vi "my_comands.vi"() -> ()   [LabVIEW 2018]
uses:
  <vilib>/Instr/_visa.llb/VISA Configure Serial Port (Instr).vi
panel:
  out "CRC16":string
  out "String":string
  in  "Array":u8[](array[numeric])=[97, 106, 241, 1, 0] format="%.0x"
  out "error out":errorcluster
  in  "baud rate (9600)":u32=9600
  in  "error in (no error)":errorcluster
  in  "VISA resource name":refnum<visa-resource-name>
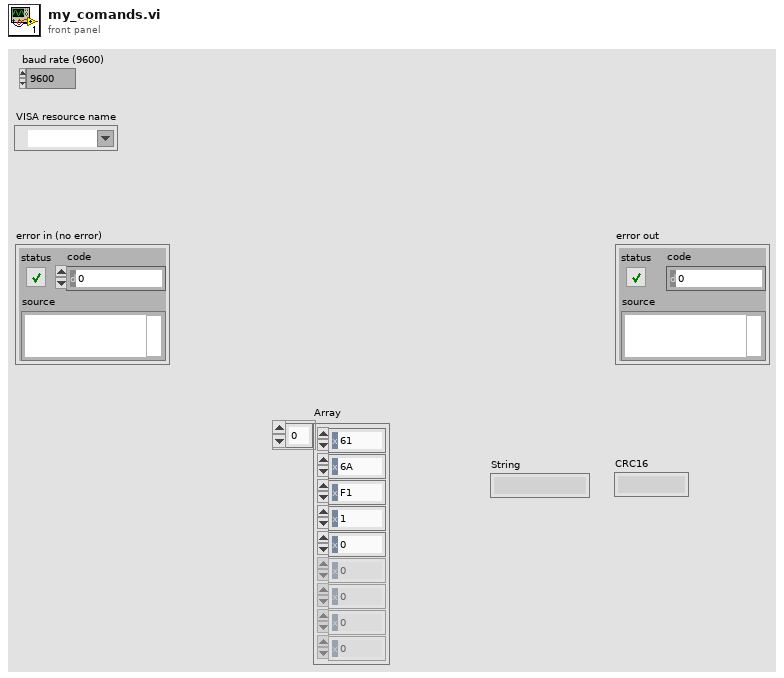
[diagram p1: front panel]
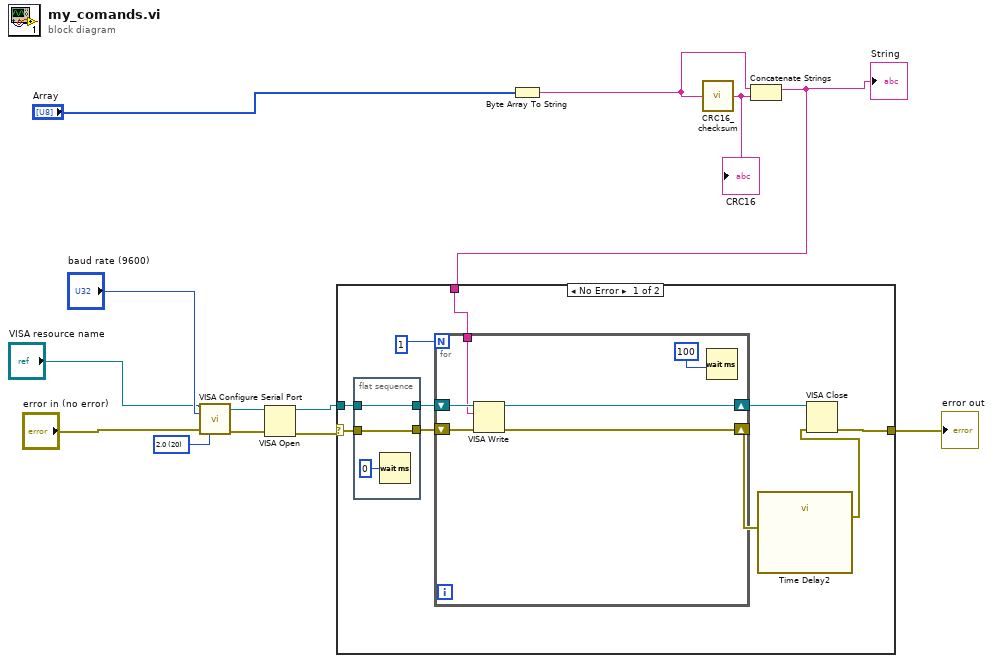
[diagram p0: block diagram]
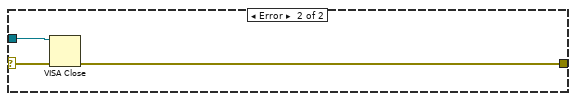
[diagram p2: hidden frame]
diagram:
  w1 = u16 20 items=["1.0"=10, "1.5"=15, "2.0"=20] ("stop bits (10: 1 bit)")
  n1 = call-poly "VISA Configure Serial Port"("VISA resource name"="VISA resource name", "baud rate (9600)"="baud rate (9600)", "error in (no error)"="error in (no error)", "stop bits (10: 1 bit)"=w1) -> ("VISA resource name out"=w3:refnum<visa-resource-name>, "error out"=w2:errorcluster)  [unwired: 10 in]
  n2 = VISA Open(error in (no error)=w2, VISA resource name=w3) -> (VISA resource name=w5:refnum<visa-resource-name>, error out=w4:errorcluster)  [unwired: 3 in]
  n3 = Byte Array To String(unsigned byte array="Array") -> (string=w8:string)
  n4 = call "CRC16_checksum.vi"("message"=w8) -> ("CRC16"=w10:string)
  "CRC16" <- w10
  n5 = Concatenate Strings(w8, w10) -> (w11:string)
  "String" <- w11
  n6 = case shown="No Error" w4 {
    selector: w4 -> [w16 w34]
    tunnel: w5 -> [w17 w35]
    tunnel: [w22 w33] -> w12
    tunnel: w11 -> [w21 _]
    frame No Error {
      n7 = flat-sequence {
        tunnel: w17 -> [w25]
        tunnel: w16 -> [w24]
        tunnel: [w24] -> w15
        tunnel: [w25] -> w14
        frame #0 {
          n8 = Wait (ms)(milliseconds to wait=u32 0) -> ()  [unwired: 1 out]
        }
      }
      n9 = for {
        N: 1 -> [_]
        shift-right: [w27] -> w19
        shift-left: w15 -> [w32]
        shift-right: [w28] -> w20
        shift-left: w14 -> [w31]
        tunnel: w21 -> [w29]
        n10 = VISA Write(VISA resource name=w31, write buffer=w29, error in (no error)=w32) -> (VISA resource name out=w28:refnum<visa-resource-name>, error out=w27:errorcluster)  [unwired: 1 out]
        n11 = Wait (ms)(milliseconds to wait=u32 100) -> ()  [unwired: 1 out]
      }
      n12 = call "Time Delay2"("error in (no error)"=w19) -> ("error out"=w18:errorcluster)  [unwired: 10 in]
      n13 = VISA Close(VISA resource name=w20, error in (no error)=w18) -> (error out=w22:errorcluster)
    }
    frame Error {
      n14 = VISA Close(VISA resource name=w35, error in (no error)=w34) -> (error out=w33:errorcluster)
    }
  }
  "error out" <- w12
